vi "gotoTopBotExp2Ronen.vi"(8 "error in (no error)":errorcluster, 9 "Distance to target":T1={"X Pos (mm)"=-2.9995918, "Y Pos (mm)"=0.610337, "Z Pos (mm)"=-0.16263409} {"Y Pos (mm)" format="%.3f"; "Z Pos (mm)" format="%.3f"; "X Pos (mm)" format="%.3f"}, 10 "motor setting":refnum<vi>, 11 "Array of all references":refnum<k7>[](array[refnum])) -> (0 "error out":errorcluster)   [LabVIEW 2014]
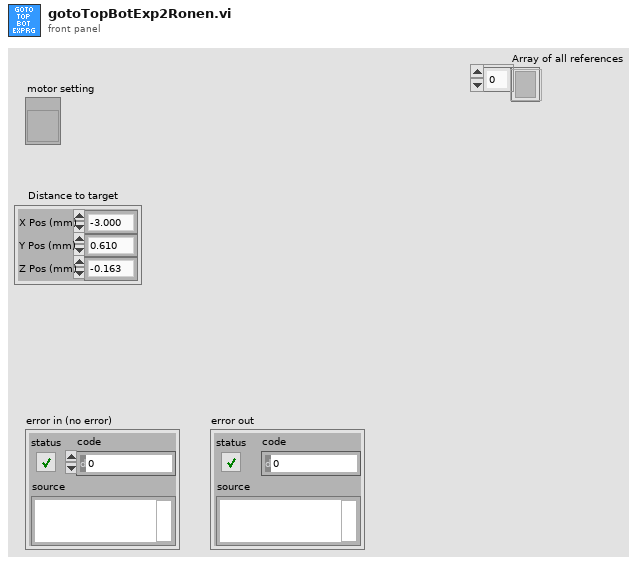
[diagram p1: front panel]
types:
  T1 = cluster{"X Pos (mm)":sgl, "Y Pos (mm)":sgl, "Z Pos (mm)":sgl}
  T2 = cluster{"X Acc (mm/s^2)":sgl, "X Vmax (mm/s)":sgl, "Y Acc (mm/s^2)":sgl, "Y Vmax (mm/s)":sgl, "Z Acc (mm/s^2)":sgl, "Z Vmax (mm/s)":sgl}
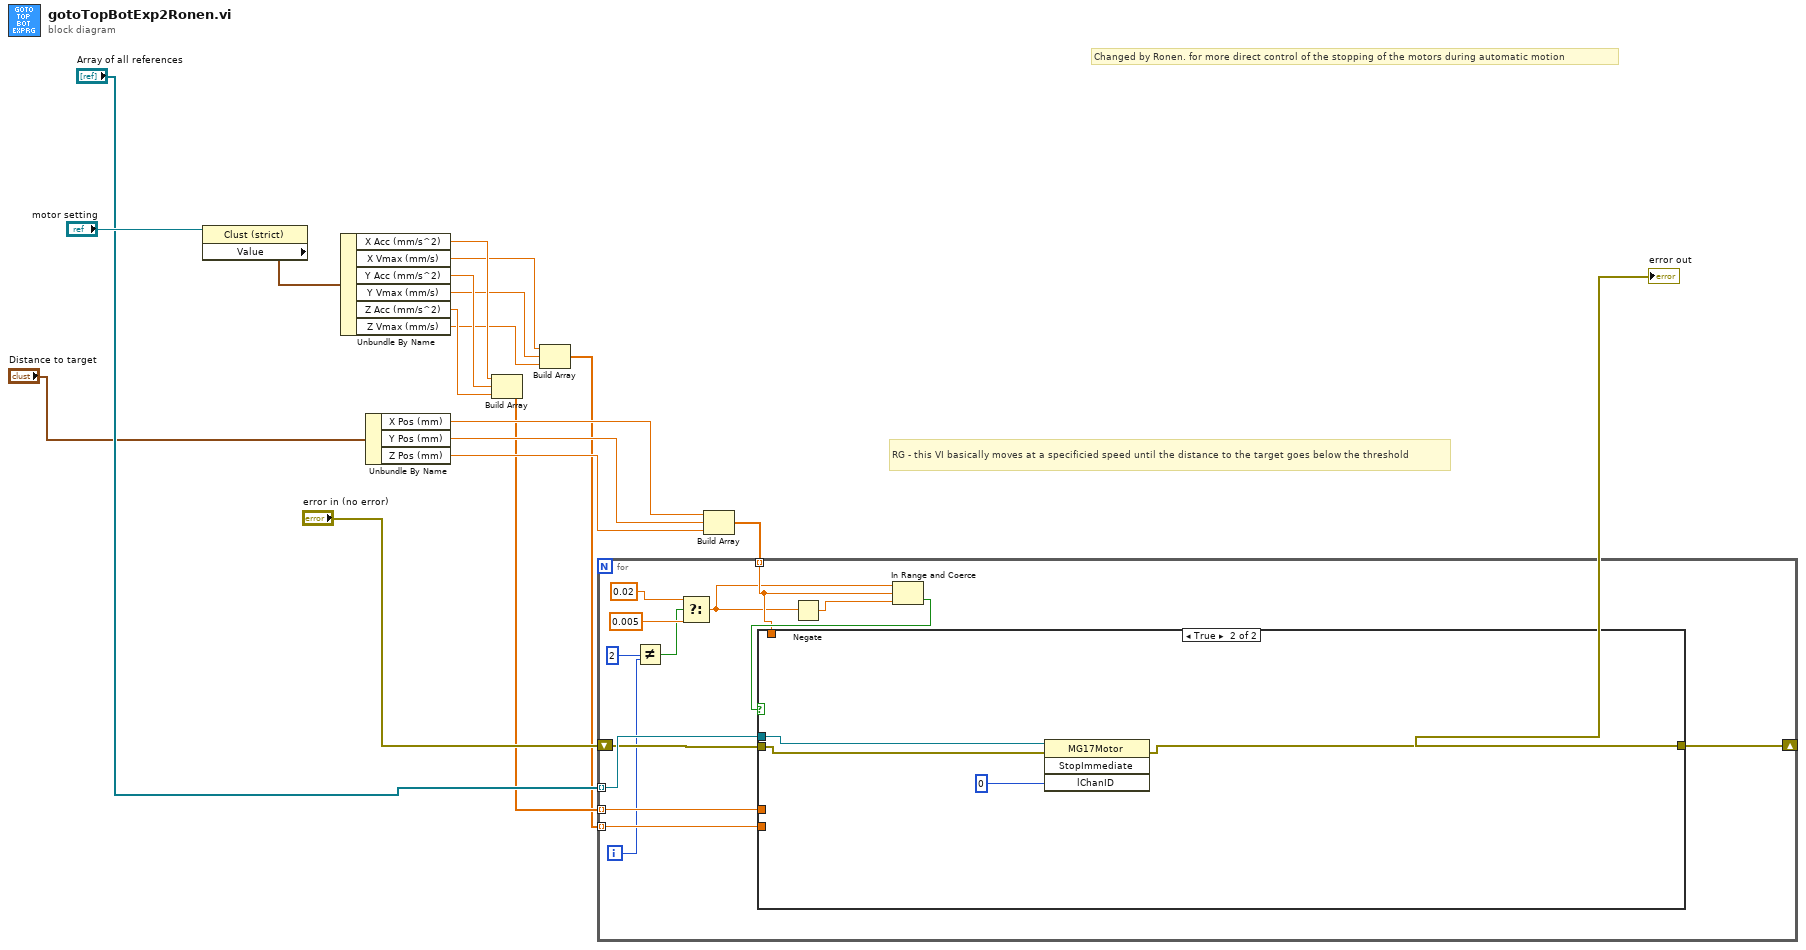
[diagram p0: block diagram]
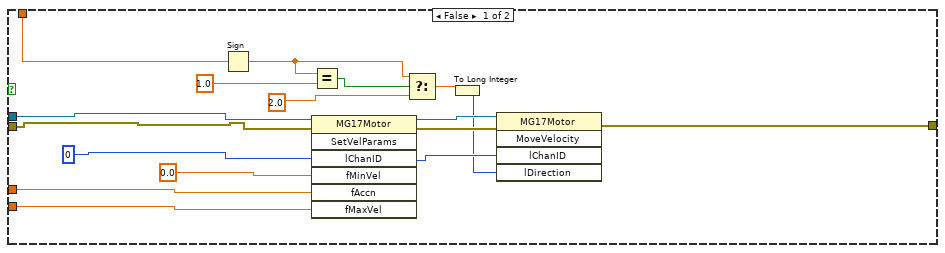
[diagram p2: hidden frame]
diagram:
  # "RG - this VI basically moves at a specificied speed until the distance to the target goes below the threshold"
  # "Changed by Ronen. for more direct control of the stopping of the motors during automatic motion"
  n1 = property on="Property Node" class="Clust (strict)"(reference="motor setting") -> ("Value"=w16:T2)  [unwired: 1 in, 2 out]
  n2 = Unbundle By Name(w16) -> ("X Acc (mm/s^2)"=w9:sgl, "X Vmax (mm/s)"=w6:sgl, "Y Acc (mm/s^2)"=w8:sgl, "Y Vmax (mm/s)"=w5:sgl, "Z Acc (mm/s^2)"=w7:sgl, "Z Vmax (mm/s)"=w4:sgl)
  n3 = Unbundle By Name("Distance to target") -> ("X Pos (mm)"=w15:sgl, "Y Pos (mm)"=w14:sgl, "Z Pos (mm)"=w13:sgl)
  n4 = Build Array(w9, w8, w7) -> (w3:sgl[])
  n5 = Build Array(w6, w5, w4) -> (w2:sgl[])
  n6 = Build Array(w15, w14, w13) -> (w11:sgl[])
  n7 = for {
    tunnel: "Array of all references" -> [w32] mode=indexing
    tunnel: w2 -> [w31] mode=indexing
    tunnel: w3 -> [w30] mode=indexing
    tunnel: w11 -> [w27] mode=indexing
    shift-right: [w29] -> w18
    shift-left: "error in (no error)" -> [w26]
    i -> [w24]
    n8 = Not Equal?(x=2, y=w24) -> (x != y?=w21:bool)
    n9 = Select(t=0.02, s=w21, f=0.005) -> (s? t:f=w20:dbl)
    n10 = Negate(x=w20) -> (-x=w19:dbl)
    n11 = In Range and Coerce(upper limit=w20, x=w27, lower limit=w19) -> (In Range?=w28:bool)  [unwired: 1 out]
    n12 = case shown="True" w28 {
      tunnel: w32 -> [w41 w53]
      tunnel: w31 -> [w48 _]
      tunnel: w30 -> [w47 _]
      tunnel: [w46 w51] -> w29
      tunnel: w27 -> [w43 _]
      tunnel: w26 -> [w40 w52]
      frame False {
        n13 = Sign(1:w43) -> (0:w38:sgl)
        n14 = Equal?(x=w38, y=1.0) -> (x = y?=w34:bool)
        n15 = invoke class="MG17Motor" method="SetVelParams"(reference=w41, error in=w40, "lChanID"=0, "fMinVel"=sgl 0.0, "fAccn"=w47, "fMaxVel"=w48) -> (reference out=w45:refnum<k7>, error out=w42:errorcluster, "lChanID"=w44:i32)  [unwired: 1 in, 4 out]
        n16 = Select(t=w38, s=w34, f=sgl 2.0 ("fMinVel")) -> (s? t:f=w36:sgl)
        n17 = To Long Integer(number=w36) -> (32bit integer=w35:i32)
        n18 = invoke class="MG17Motor" method="MoveVelocity"(reference=w45, error in=w42, "lChanID"=w44, "lDirection"=w35) -> (error out=w46:errorcluster)  [unwired: 1 in, 4 out]
      }
      frame True {
        n19 = invoke class="MG17Motor" method="StopImmediate"(reference=w53, error in=w52, "lChanID"=0) -> (error out=w51:errorcluster)  [unwired: 1 in, 3 out]
      }
    }
  }
  "error out" <- w18
